vi "LR-Determine-zero.vi"(7 "Zero level settings":T2, 8 "error in (no error)":errorcluster, 9 "Power in":dbl[](array[numeric]), 11 "Results in":T1) -> (0 "error out":errorcluster, 1 "Power":dbl[](array[numeric]), 3 "Results":T1, 4 "Valid?":bool)   [LabVIEW 2013, in "HardwareCharacterization.lvlib" / "HC-LaserResponse.lvclass"]
doc: "Use this template to build a VI to use as a subVI."
uses:
  HC-LaserResponse.lvclass
  Settings-zero.ctl
  Test-results.ctl
  <vilib>/Analysis/baseanly.llb/Mean (DBL).vi
  <vilib>/Analysis/NI_AALBase.lvlib
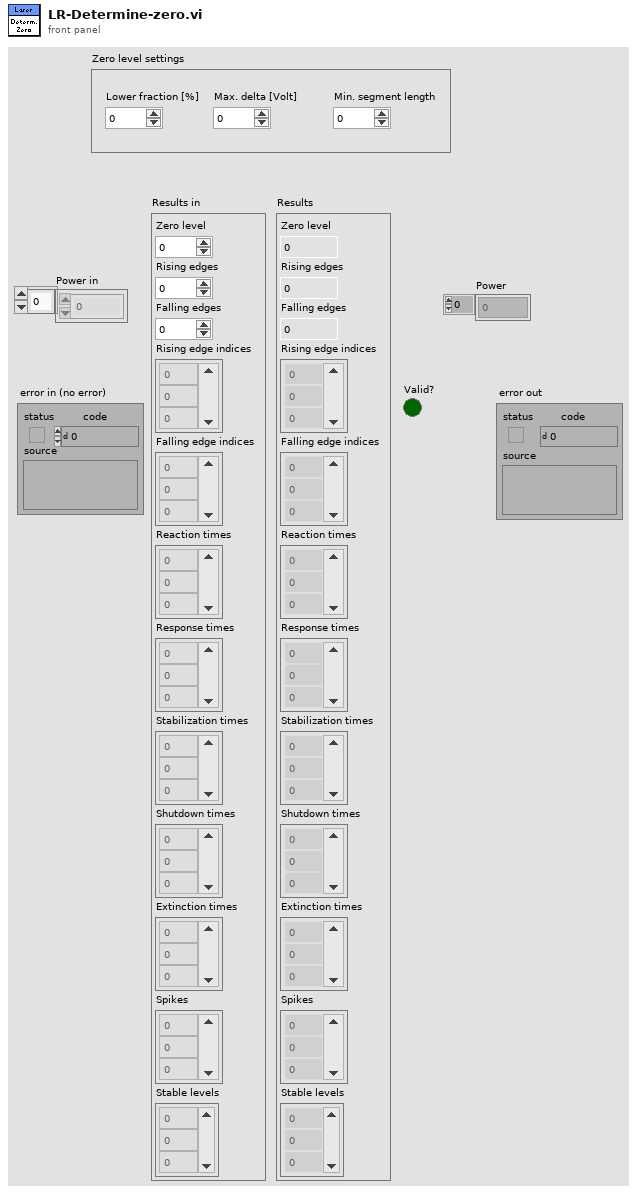
[diagram p1: front panel]
types:
  T1 = typedef "HardwareCharacterization.lvlib/HC-LaserResponse.lvclass/Test-results.ctl" = cluster{"Zero level":dbl, "Rising edges":i32, "Falling edges":i32, "Rising edge indices":dbl[], "Falling edge indices":dbl[], "Reaction times":dbl[], "Response times":dbl[], "Stabilization times":dbl[], "Shutdown times":dbl[], "Extinction times":dbl[], "Spikes":i32[], "Stable levels":dbl[]}
  T2 = typedef "HardwareCharacterization.lvlib/HC-LaserResponse.lvclass/Settings-zero.ctl" = cluster{"Lower fraction [%]":i32, "Max. delta [Volt]":dbl, "Min. segment length":i32}
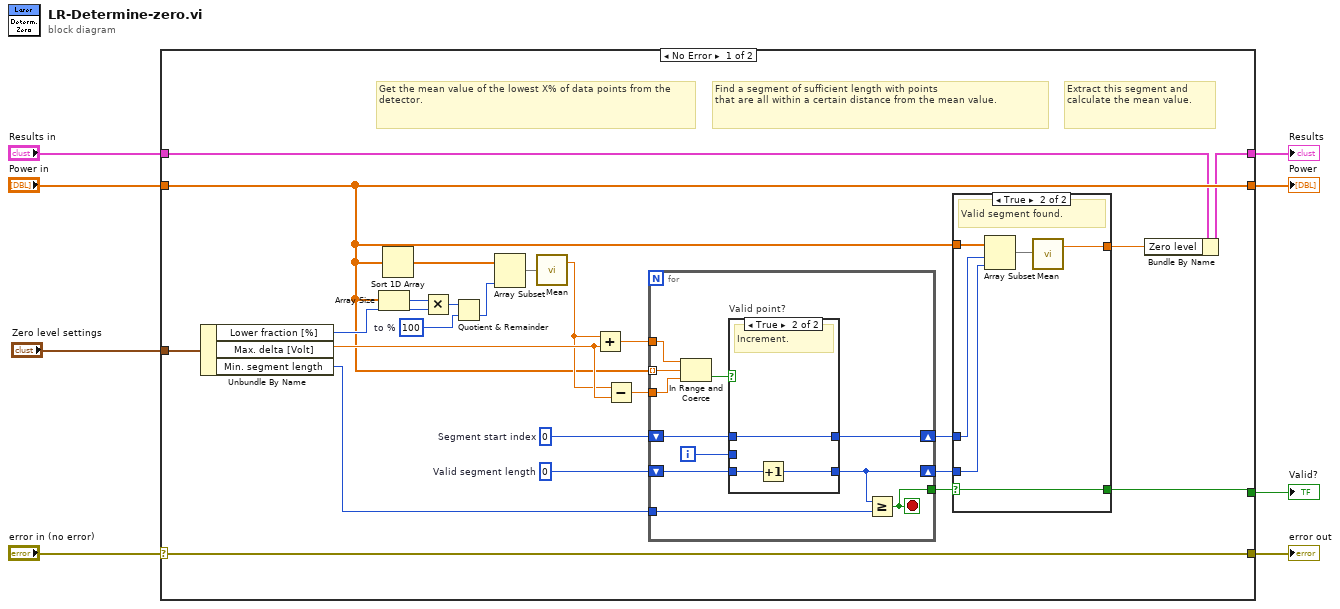
[diagram p0: block diagram]
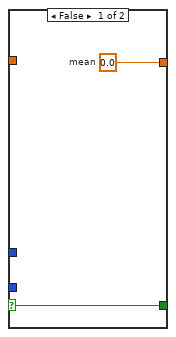
[diagram p2: hidden frame]
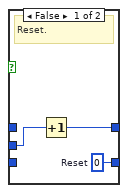
[diagram p3: hidden frame]
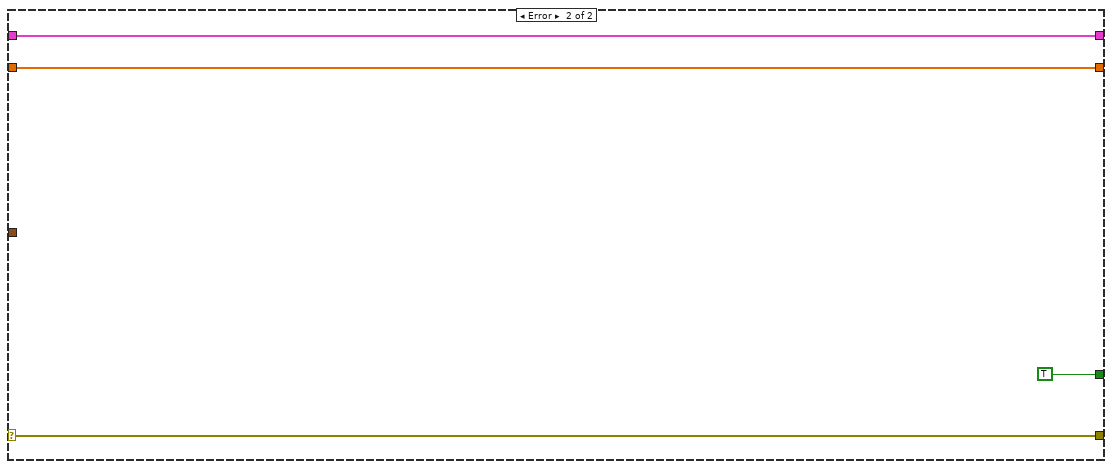
[diagram p4: hidden frame]
diagram:
  n1 = case shown="No Error" "error in (no error)" {
    selector: "error in (no error)" -> [w21 w61]
    tunnel: [w21 w61] -> w7
    tunnel: "Zero level settings" -> [w32 _]
    tunnel: [w17 TRUE] -> w5
    tunnel: "Power in" -> [w12 w59]
    tunnel: [w12 w59] -> w3
    tunnel: "Results in" -> [w11 w58]
    tunnel: [w10 w58] -> w1
    frame No Error {
      w22 = 0  # Segment start index
      w28 = 0  # Valid segment length
      w13 = 100  # to %
      # "Extract this segment and \ncalculate the mean value."
      # "Find a segment of sufficient length with points \nthat are all within a certain distance from the mean value."
      # "Get the mean value of the lowest X% of data points from the detector."
      n2 = Unbundle By Name(w32) -> ("Lower fraction [%]"=w14:i32, "Max. delta [Volt]"=w24:dbl, "Min. segment length"=w27:i32)
      n3 = Array Size(array=w12) -> (size(s)=w30:i32)
      n4 = Sort 1D Array(array=w12) -> (sorted array=w31:dbl[])
      n5 = Multiply(x=w30, y=w14) -> (x*y=w29:i32)
      n6 = Quotient & Remainder(x=w29, y=w13) -> (floor(x/y)=w16:i32)  [unwired: 1 out]
      n7 = Array Subset(array=w31, length=w16) -> (w23:dbl[])  [unwired: 1 in]
      n8 = call-poly <vilib>:"Mean.vi"("X"=w23) -> ("mean"=w15:dbl)  [unwired: 1 out]
      n9 = Add(x=w15, y=w24) -> (x+y=w26:dbl)
      n10 = Subtract(x=w15, y=w24) -> (x-y=w25:dbl)
      n11 = for {
        shift-right: [w42] -> w20
        shift-left: w28 -> [w47]
        tunnel: w27 -> [w43]
        tunnel: w26 -> [w50]
        tunnel: w25 -> [w49]
        tunnel: w12 -> [w51] mode=indexing
        shift-right: [w44] -> w18
        shift-left: w22 -> [w45]
        tunnel: [w41] -> w19
        i -> [w46]
        stop <- w41 stop-if-true
        n12 = In Range and Coerce(upper limit=w50, x=w51, lower limit=w49) -> (In Range?=w48:bool)  [unwired: 1 out]
        n13 = case "Valid point?" shown="True" w48 {
          tunnel: w47 -> [_ w57]
          tunnel: [w54 w56] -> w42
          tunnel: w46 -> [w53 _]
          tunnel: w45 -> [_ w55]
          tunnel: [w52 w55] -> w44
          frame False {
            w54 = 0  # Reset
            # "Reset."
            n14 = Increment(x=w53) -> (x+1=w52:i32)
          }
          frame True {
            # "Increment."
            n15 = Increment(x=w57) -> (x+1=w56:i32)
          }
        }
        n16 = Greater Or Equal?(x=w42, y=w43) -> (x >= y?=w41:bool)
      }
      n17 = case shown="True" w19 {
        selector: w19 -> [w33 w35]
        tunnel: w20 -> [_ w40]
        tunnel: w12 -> [_ w39]
        tunnel: w18 -> [_ w38]
        tunnel: [w34 w36] -> w9
        tunnel: [w33 w35] -> w17
        frame False {
          w34 = 0.0  # mean
        }
        frame True {
          # "Valid segment found."
          n18 = Array Subset(array=w39, index=w38, length=w40) -> (w37:dbl[])
          n19 = call-poly <vilib>:"Mean.vi"("X"=w37) -> ("mean"=w36:dbl)  [unwired: 1 out]
        }
      }
      n20 = Bundle By Name(cluster=w11, "Zero level"=w9) -> (w10:T1)
    }
    frame Error {
    }
  }
  "error out" <- w7
  "Valid?" <- w5
  "Power" <- w3
  "Results" <- w1
